vi "Move servo.vi"(8 "Duty Cycle":dbl format="%.6f", 10 "Output Terminal":tag="/Dev1/PFI3", 11 "Counter":tag="Dev1/ctr0") -> (0 "Actual Duty Cycle":dbl)   [LabVIEW 2017]
uses:
  <vilib>/Utility/error.llb/DialogType.ctl
  <vilib>/DAQmx/create/channels.llb/DAQmx Create Channel (CO-Pulse Generation-Frequency).vi
  <vilib>/DAQmx/configure/timing.llb/DAQmx Timing (Implicit).vi
  <resource>/objmgr/daqmx.rc
panel:
  in  "Stop":bool
  # "Channel Settings"
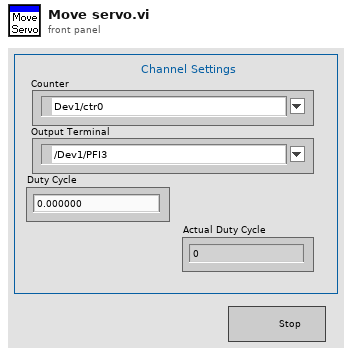
[diagram p1: front panel]
types:
  T1 = typedef "DialogType.ctl" = u16
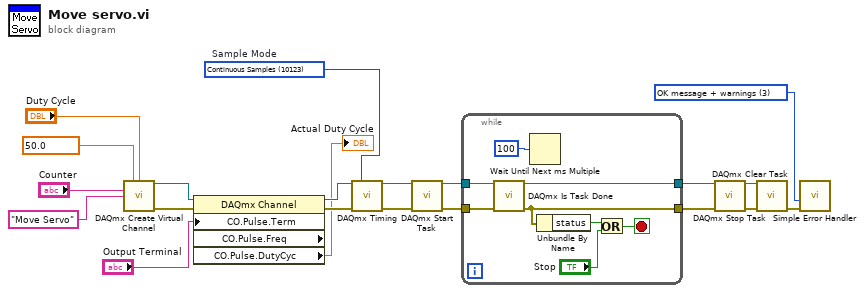
[diagram p0: block diagram]
diagram:
  w4 = 10123 items=["Finite Samples"=10178, "Continuous Samples"=10123, "Hardware Timed Single Point"=12522]  # Sample Mode
  w12 = T1 3 items=["no dialog", "OK message", "continue or stop message", "OK message + warnings", "continue/stop + warnings"] ("type of dialog (OK msg:1)")
  n1 = call-poly <vilib>:"DAQmx Create Virtual Channel.vi"("frequency"=50.0 ("Frequency"), "duty cycle"="Duty Cycle", "counter"="Counter", "name to assign"="Move Servo") -> ("task out"=w10:refnum<k21>, "error out"=w9:errorcluster)  [unwired: 10 in]
  n2 = property class="DAQmx Channel" props=["CO.Pulse.Term", "CO.Pulse.Freq", "CO.Pulse.DutyCyc"](reference=w10, error in=w9, "CO.Pulse.Term"="Output Terminal") -> (reference out=w20:refnum<k21>, error out=w21:errorcluster, "CO.Pulse.DutyCyc"=→"Actual Duty Cycle":dbl)  [unwired: 1 out]
  n3 = call-poly <vilib>:"DAQmx Timing.vi"("task/channels in"=w20, "sample mode"=w4, "error in"=w21) -> ("task out"=w19:refnum<k21>, "error out"=w18:errorcluster)  [unwired: 11 in]
  n4 = call <vilib>:"DAQmx Start Task.vi"("task/channels in"=w19, "error in"=w18) -> ("task out"=w2:refnum<k21>, "error out"=w3:errorcluster)  [unwired: 12 in]
  n5 = while {
    tunnel: w2 -> [w29]
    tunnel: w3 -> [w28]
    tunnel: [w23] -> w14
    tunnel: [w22] -> w13
    stop <- w27 stop-if-true
    n6 = call <vilib>:"DAQmx Is Task Done.vi"("task/channels in"=w29, "error in"=w28) -> ("task out"=w23:refnum<k21>, "error out"=w22:errorcluster)  [unwired: 11 in, 1 out]
    n7 = Wait Until Next ms Multiple(millisecond multiple=u32 100) -> ()  [unwired: 1 out]
    n8 = Unbundle By Name(w22) -> ("status"=w26:bool)
    n9 = Or(x=w26, y="Stop") -> (x .or. y?=w27:bool)
  }
  n10 = call <vilib>:"DAQmx Stop Task.vi"("task/channels in"=w14, "error in"=w13) -> ("task out"=w16:refnum<k21>, "error out"=w15:errorcluster)  [unwired: 12 in]
  n11 = call <vilib>:"DAQmx Clear Task.vi"("task in"=w16, "error in"=w15) -> ("error out"=w17:errorcluster)  [unwired: 13 in]
  n12 = call <vilib>:"Simple Error Handler.vi"("type of dialog (OK msg:1)"=w12, "error in (no error)"=w17) -> ()  [unwired: 3 in, 5 out]
